vi "Commit Calibration Data.vi"(0 "CART TCP Connection In":refnum<k5>, 11 "error in (no error)":errorcluster) -> (4 "CART TCP Connection Out":refnum<k5>, 8 "TCP Messages":string[](array[string]), 15 "error out":errorcluster)   [LabVIEW 2011]
uses:
  WLAN/UUT/QCA/NART Constants.vi
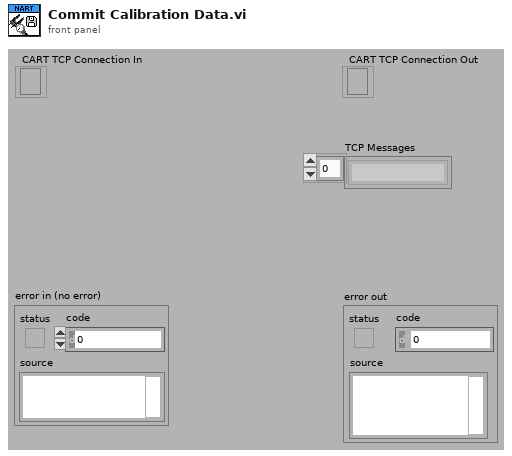
[diagram p1: front panel]
types:
  T1 = cluster{"Name":string, "Type":enum16{"decimal", "string", "float", "hex"}}[]
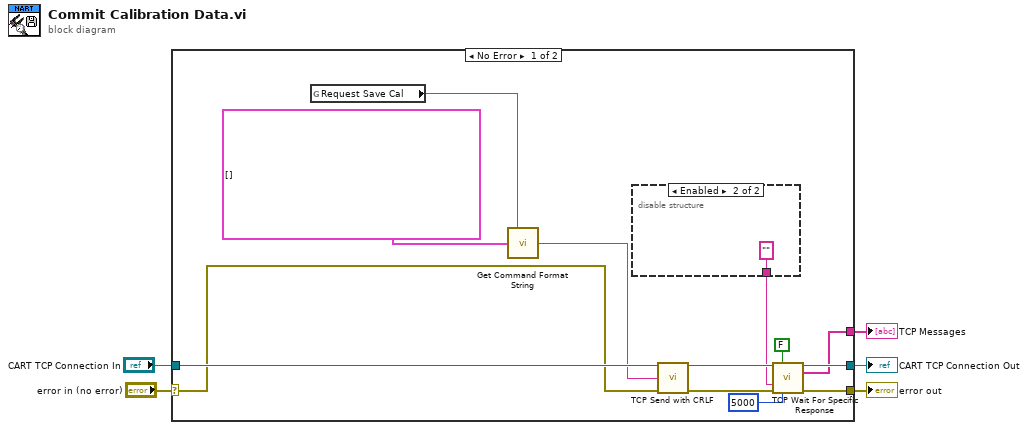
[diagram p0: block diagram]
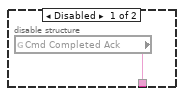
[diagram p2: hidden frame]
diagram:
  n1 = case shown="No Error" "error in (no error)" {
    selector: "error in (no error)" -> [w15 w22]
    tunnel: [w12 w22] -> w4
    tunnel: "CART TCP Connection In" -> [w18 w21]
    tunnel: [w13 w21] -> w2
    tunnel: [w9 _] -> w1
    frame No Error {
      n2 = global read "NART Constants.vi" "Request Save Cal"() -> (w7:string)
      n3 = call "Get Command Format String.vi"("Command"=w7, "Parameters"=T1 []) -> ("Command Format String"=w16:string)  [unwired: 13 in]
      n4 = disable-structure shown="Enabled" {
        disable-tunnel: [w19 "" ("Expected Message Start (\"\":any)")] -> w6
        frame Disabled {
          n5 = global read "NART Constants.vi" "Cmd Completed Ack"() -> (w19:string)
        }
        frame Enabled {
        }
      }
      n6 = call "TCP Send with CRLF.vi"("CART TCP Connection"=w18, "data in"=w16, "error IO"=w15) -> ("CART TCP Connection Out"=w14:refnum<k5>, "error out"=w11:errorcluster)  [unwired: 11 in]
      n7 = call "TCP Wait For Specific Response.vi"("TCP Connection In"=w14, "Next response (t)"=FALSE, "Expected Message Start (\"\":any)"=w6, "error in"=w11, "Timeout (250 ms)"=5000) -> ("TCP Connection Out"=w13:refnum<k5>, "TCP Messages"=w9:string[], "error out"=w12:errorcluster)  [unwired: 7 in, 1 out]
    }
    frame Error {
    }
  }
  "error out" <- w4
  "CART TCP Connection Out" <- w2
  "TCP Messages" <- w1
